vi "SUB-Graph plot select.vi"(3 "CDC(PCAP02) Graph 2":refnum<vi>) -> ()   [LabVIEW 2015]
doc: "Use this template to create an application that executes repeatedly until you click the Stop button. This template polls the state of the Stop button and does not use events. Use the Top-Level Application template (not available in the Base package) to create a single-loop application with event handling."
panel:
  in  "All Raw":bool
  in  "All Normal":bool
  in  "All Off":bool
  in  "All On":bool
  in  "Plot List":cluster{"Plot Name":string, "Select":bool}[](array[cluster])=[{"Plot Name"="Left Wing-A", "Select"=TRUE}, {"Plot Name"="Left Wing-B", "Select"=TRUE}, {"Plot Name"="Left Wing-C", "Select"=TRUE}, {"Plot Name"="Right Wing-A", "Select"=TRUE}, {"Plot Name"="Right Wing-B", "Select"=TRUE}, {"Plot Name"="Right Wing-C", "Select"=TRUE}, {"Plot Name"="(Raw)LW-A", "Select"=TRUE}, {"Plot Name"="(Raw)LW-B", "Select"=TRUE}, {"Plot Name"="(Raw)LW-C", "Select"=TRUE}, {"Plot Name"="(Raw)RW-A", "Select"=TRUE}, {"Plot Name"="(Raw)RW-B", "Select"=TRUE}, {"Plot Name"="(Raw)RW-C", "Select"=TRUE}]
  out "Update?":bool=TRUE
  in  "Cancel":bool
  in  "OK":bool
  # "[Graph] Plot On/Off selection"
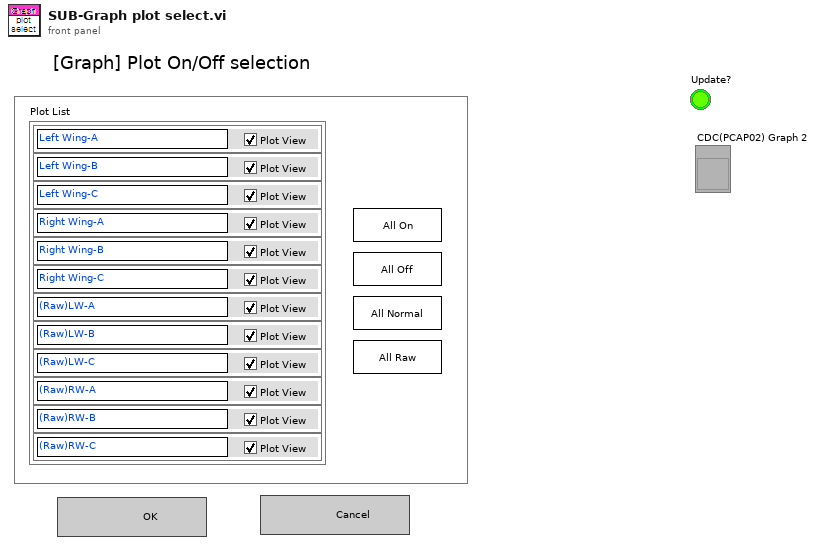
[diagram p1: front panel]
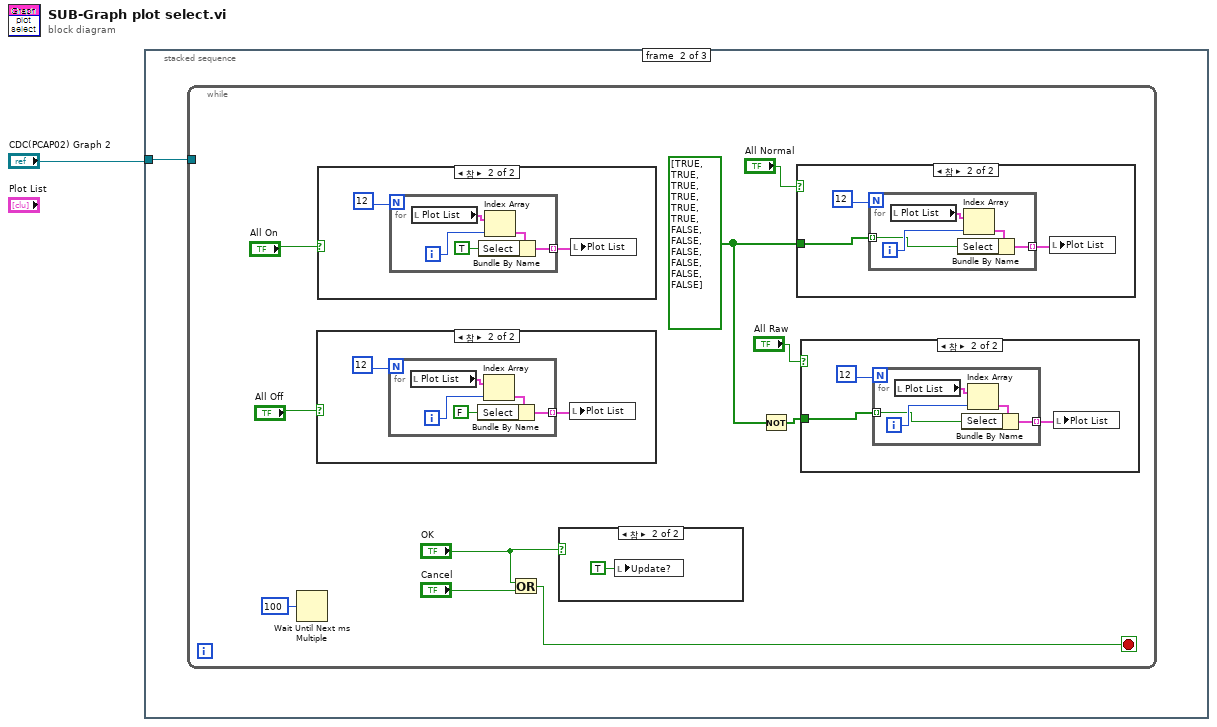
[diagram p0: block diagram]
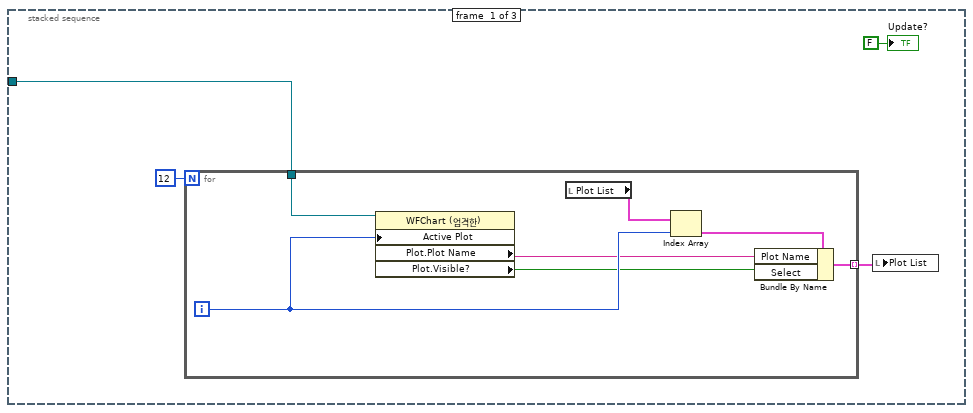
[diagram p2: hidden frame]
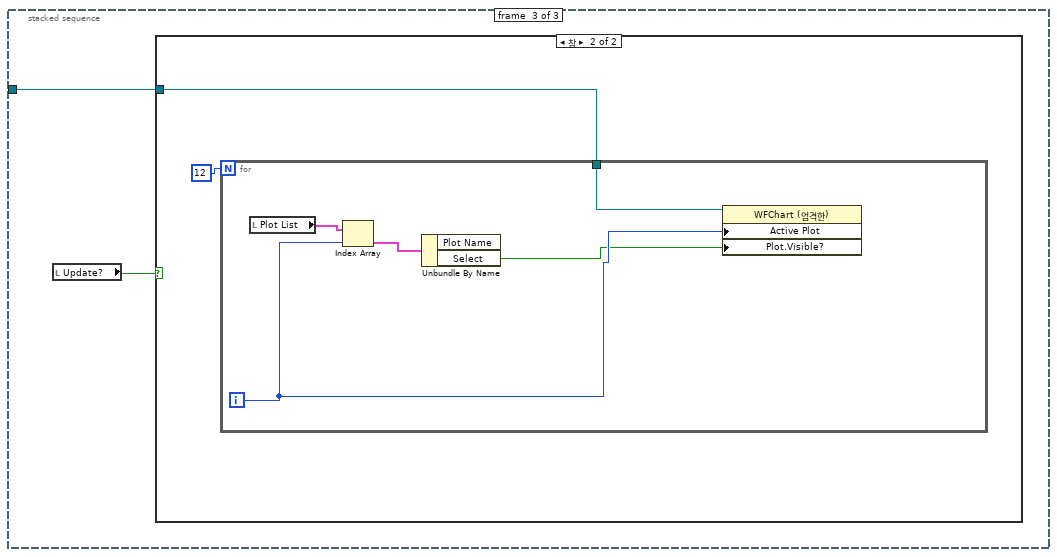
[diagram p8: hidden frame]
diagram:
  n1 = stacked-sequence {
    tunnel: "CDC(PCAP02) Graph 2" -> [w3 w13 w55]
    frame #0 {
      n2 = for {
        N: 12 -> [_]
        tunnel: [w7] -> w5 mode=indexing
        tunnel: w3 -> [w6]
        i -> [w11]
        n3 = property class="WFChart (엄격한)"(reference=w6, "Active Plot"=w11) -> ("Plot.Plot Name"=w9:string, "Plot.Visible?"=w8:bool)  [unwired: 1 in, 2 out]
        n4 = local read "Plot List"() -> (w12:cluster{"Plot Name":string, "Select":bool}[])
        n5 = Index Array(array=w12, index=w11) -> (element=w10:cluster{"Plot Name":string, "Select":bool})
        n6 = Bundle By Name(cluster=w10, "Plot Name"=w9, "Select"=w8) -> (w7:cluster{"Plot Name":string, "Select":bool})
      }
      n7 = local write "Plot List"(w5) -> ()
      "Update?" <- FALSE ("Update?")
    }
    frame #1 {
      n8 = while {
        tunnel: w13 -> [_]
        stop <- w20 stop-if-true
        w14 = bool[] [TRUE, TRUE, TRUE, TRUE, TRUE, TRUE, FALSE, FALSE, FALSE, FALSE, FALSE, FALSE] ("Select")
        n9 = Wait Until Next ms Multiple(millisecond multiple=u32 100 ("ms 배수")) -> ()  [unwired: 1 out]
        n10 = case shown="참" "All Off" {
          frame False {
          }
          frame True {
            n11 = for {
              N: 12 -> [_]
              tunnel: [w43] -> w40 mode=indexing
              i -> [w45]
              n12 = local read "Plot List"() -> (w46:cluster{"Plot Name":string, "Select":bool}[])
              n13 = Index Array(array=w46, index=w45) -> (element=w44:cluster{"Plot Name":string, "Select":bool})
              n14 = Bundle By Name(cluster=w44, "Select"=FALSE) -> (w43:cluster{"Plot Name":string, "Select":bool})
            }
            n15 = local write "Plot List"(w40) -> ()
          }
        }
        n16 = case shown="참" "All On" {
          frame False {
          }
          frame True {
            n17 = for {
              N: 12 -> [_]
              tunnel: [w50] -> w48 mode=indexing
              i -> [w52]
              n18 = local read "Plot List"() -> (w53:cluster{"Plot Name":string, "Select":bool}[])
              n19 = Index Array(array=w53, index=w52) -> (element=w51:cluster{"Plot Name":string, "Select":bool})
              n20 = Bundle By Name(cluster=w51, "Select"=TRUE) -> (w50:cluster{"Plot Name":string, "Select":bool})
            }
            n21 = local write "Plot List"(w48) -> ()
          }
        }
        n22 = Or(x="OK", y="Cancel") -> (x .or. y?=w20:bool)
        n23 = case shown="참" "OK" {
          frame False {
          }
          frame True {
            n24 = local write "Update?"(TRUE ("Update?")) -> ()
          }
        }
        n25 = Not(x=w14) -> (.not. x?=w15:bool[])
        n26 = case shown="참" "All Normal" {
          tunnel: w14 -> [_ w32]
          frame False {
          }
          frame True {
            n27 = for {
              N: 12 -> [_]
              tunnel: [w36] -> w34 mode=indexing
              tunnel: w32 -> [w35] mode=indexing
              i -> [w38]
              n28 = local read "Plot List"() -> (w39:cluster{"Plot Name":string, "Select":bool}[])
              n29 = Index Array(array=w39, index=w38) -> (element=w37:cluster{"Plot Name":string, "Select":bool})
              n30 = Bundle By Name(cluster=w37, "Select"=w35) -> (w36:cluster{"Plot Name":string, "Select":bool})
            }
            n31 = local write "Plot List"(w34) -> ()
          }
        }
        n32 = case shown="참" "All Raw" {
          tunnel: w15 -> [_ w24]
          frame False {
          }
          frame True {
            n33 = for {
              N: 12 -> [_]
              tunnel: [w28] -> w26 mode=indexing
              tunnel: w24 -> [w27] mode=indexing
              i -> [w30]
              n34 = local read "Plot List"() -> (w31:cluster{"Plot Name":string, "Select":bool}[])
              n35 = Index Array(array=w31, index=w30) -> (element=w29:cluster{"Plot Name":string, "Select":bool})
              n36 = Bundle By Name(cluster=w29, "Select"=w27) -> (w28:cluster{"Plot Name":string, "Select":bool})
            }
            n37 = local write "Plot List"(w26) -> ()
          }
        }
      }
    }
    frame #2 {
      n38 = local read "Update?"() -> (w56:bool)
      n39 = case shown="참" w56 {
        tunnel: w55 -> [_ w57]
        frame False {
        }
        frame True {
          n40 = for {
            N: 12 -> [_]
            tunnel: w57 -> [w61]
            i -> [w60]
            n41 = local read "Plot List"() -> (w63:cluster{"Plot Name":string, "Select":bool}[])
            n42 = Index Array(array=w63, index=w60) -> (element=w62:cluster{"Plot Name":string, "Select":bool})
            n43 = Unbundle By Name(w62) -> ("Select"=w59:bool)  [unwired: 1 out]
            n44 = property class="WFChart (엄격한)"(reference=w61, "Active Plot"=w60, "Plot.Visible?"=w59) -> ()  [unwired: 1 in, 2 out]
          }
        }
      }
    }
  }
